vi "Test Create Complex Number To String.vi"() -> ()   [LabVIEW 2014]
uses:
  <vilib>/Aledyne-TSXperts/Arduino Compatible Compiler for LabVIEW/addons/Complex Numbers/Complex Numbers.lvlib
panel:
  out "Error Out":errorcluster
  in  "Error In":errorcluster
  out "String complex num.":string
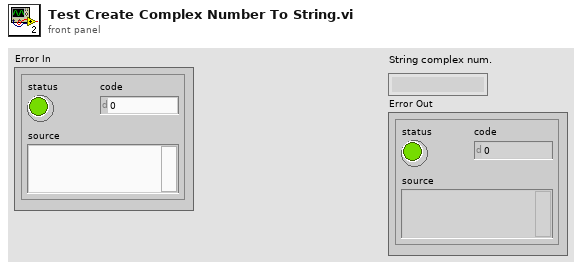
[diagram p1: front panel]
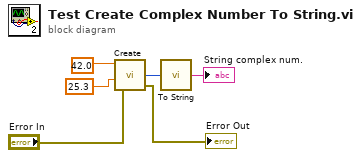
[diagram p0: block diagram]
diagram:
  n1 = call <vilib>:"Create.vi"("Error In"="Error In", "Imag"=25.3, "Real"=42.0) -> ("Error Out"=→"Error Out":errorcluster, "Complex"=w5:u32)  [unwired: 2 in]
  n2 = call <vilib>:"To String.vi"("Complex number"=w5) -> ("String complex num."=→"String complex num.":string)
